vi "Test.vi"() -> ()   [LabVIEW 2012]
uses:
  Multi Segment Waveform.xctl
panel:
  out "Y":dbl[](array[numeric])
  in  "Rate Mode":bool
  in  "Multi Segment Waveform":waveform(dbl)(xcontrol)
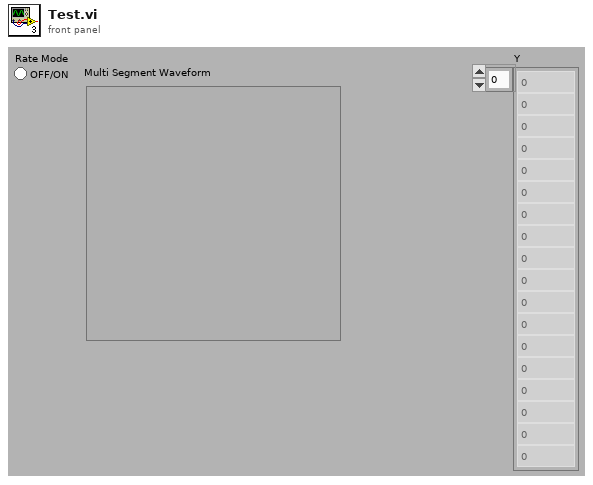
[diagram p1: front panel]
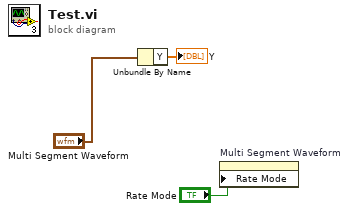
[diagram p0: block diagram]
diagram:
  n1 = Unbundle By Name("Multi Segment Waveform") -> ("Y"=→"Y":dbl[])
  n2 = property on="Multi Segment Waveform" class="Multi Segment Waveform (strict)"("Rate Mode"="Rate Mode") -> ()  [unwired: 2 in, 2 out]
